vi "get parameter - i16.vi"(8 "error in (no error)":errorcluster, 10 "parameter":u8 format="%x", 11 "channel":u16 format="%x") -> (0 "error out":errorcluster, 3 "value":i16)   [LabVIEW 2024, in "atsj peakcan basic.lvlib"]
doc: "Gets a parameter from a PeakCAN <b>channel</b>."
uses:
  atsj peakcan basic.lvlib
  support/x64/PCANBasic.dll
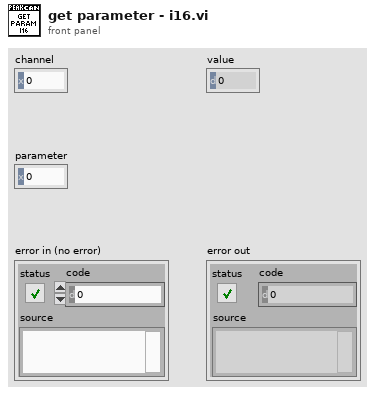
[diagram p1: front panel]
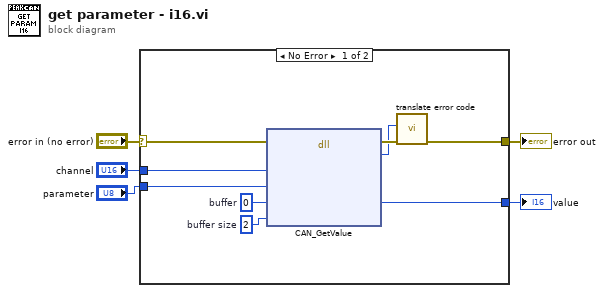
[diagram p0: block diagram]
diagram:
  n1 = case shown="No Error" "error in (no error)" {
    selector: "error in (no error)" -> [w10 w15]
    tunnel: [w9 w15] -> w4
    tunnel: [w8 _] -> w3
    tunnel: "channel" -> [w7 _]
    tunnel: "parameter" -> [w6 _]
    frame No Error {
      w14 = u16 2  # buffer size
      w13 = i16 0  # buffer
      n2 = dll-call lib="C:/atsj/plateau/atsj-peakcan-basic-for-labview/src/support/x64/PCANBasic.dll" fn="CAN_GetValue" ("get parameter - i16")(error in=w10, "Channel"=w7, "Parameter"=w6, "Buffer"=w13, "BufferLength"=w14) -> (error out=w12:errorcluster, "Status"=w11:u32, "Buffer"=w8:i16)  [unwired: 5 in, 1 out]
      n3 = call "translate error code.vi"("error in (no error)"=w12, "error code"=w11) -> ("error out"=w9:errorcluster)  [unwired: 9 in]
    }
    frame Error {
    }
  }
  "error out" <- w4
  "value" <- w3
